vi "MotionProfile.vi"() -> ()   [LabVIEW 2016]
uses:
  <vilib>/Analysis/polynomials.llb/Polynomial Plot (Range).vi
  <vilib>/Analysis/polynomials.llb/nth Derivative of Polynomial (DBL).vi
  <vilib>/Analysis/NI_AALPro.lvlib
  <vilib>/addons/control/pid/NI_PID_pid.lvlib
panel:
  in  "Curve Constraints":cluster{"Orientiation Control":dbl, "Alpha":dbl}
  in  "Motion Constraints":T1={"Time Resolution (ms)"=10, "Max Acceleration"=40.0, "Cruising Velocity"=20.0}
  out "XY Graph 2":cluster{"X":dbl, "Y":dbl}[](graph)
  out "XY Graph":cluster{"X":dbl, "Y":dbl}[](graph)
  out "Corrected Motion Cluster":T2(array[cluster])
  in  "Velocity":dbl[](array[numeric])
  in  "Heading":dbl[](array[numeric])
  in  "X":dbl[](array[numeric])
  in  "Y":dbl[](array[numeric])
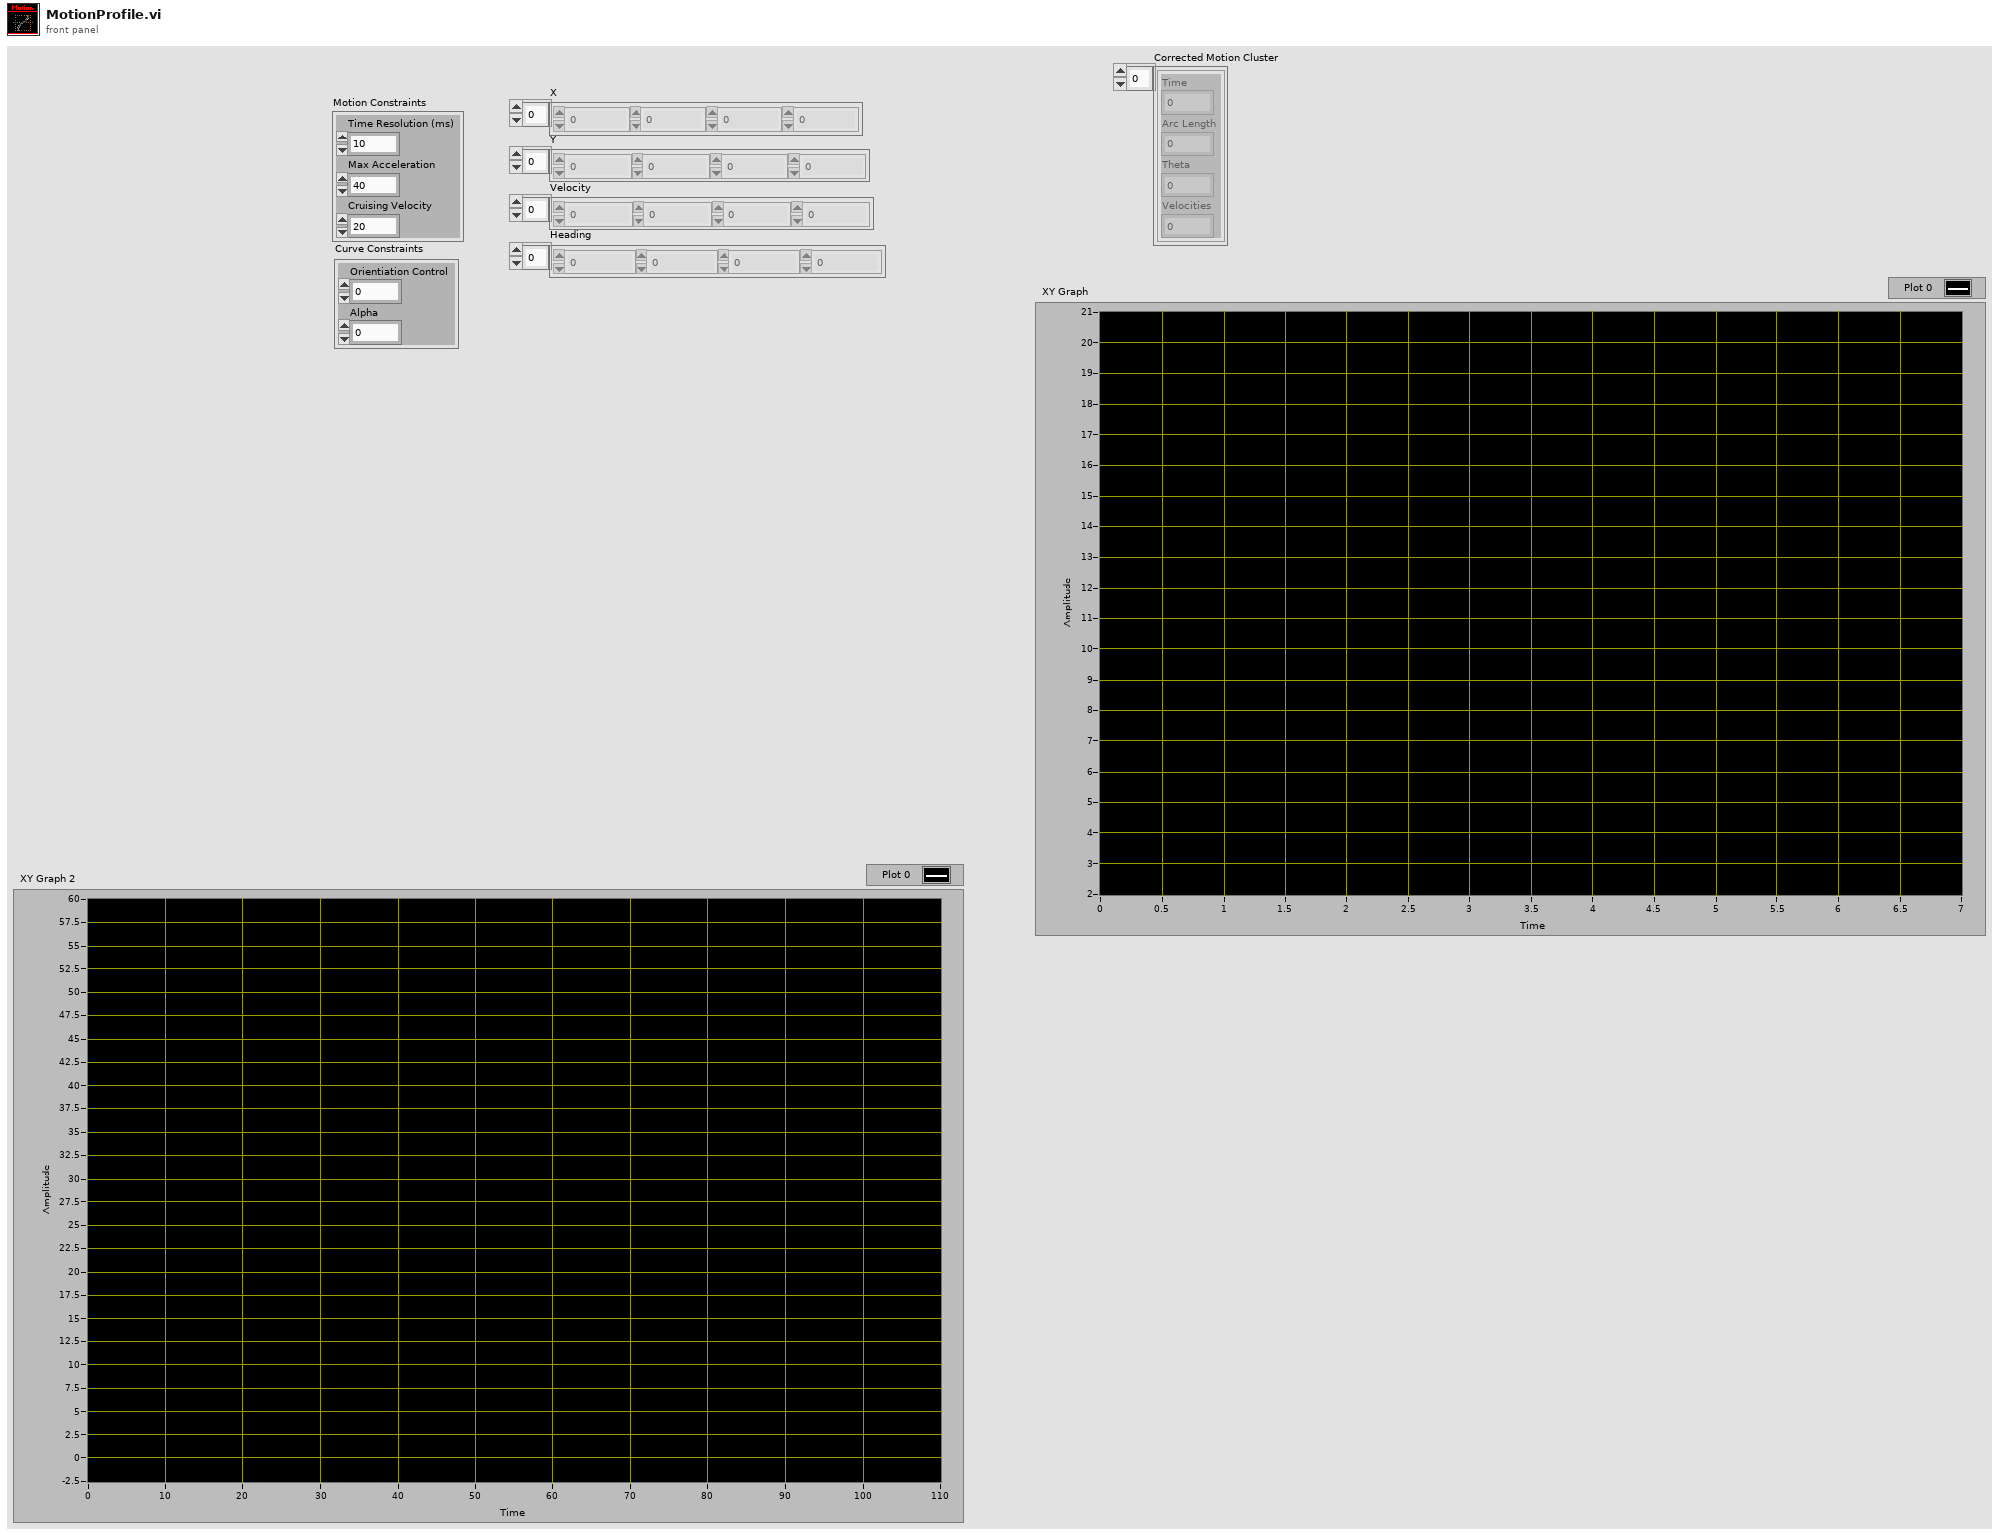
[diagram p1: front panel]
types:
  T1 = cluster{"Time Resolution (ms)":i32, "Max Acceleration":dbl, "Cruising Velocity":dbl}
  T2 = cluster{"Time":dbl, "Arc Length":dbl, "Theta":dbl, "Velocities":dbl}[]
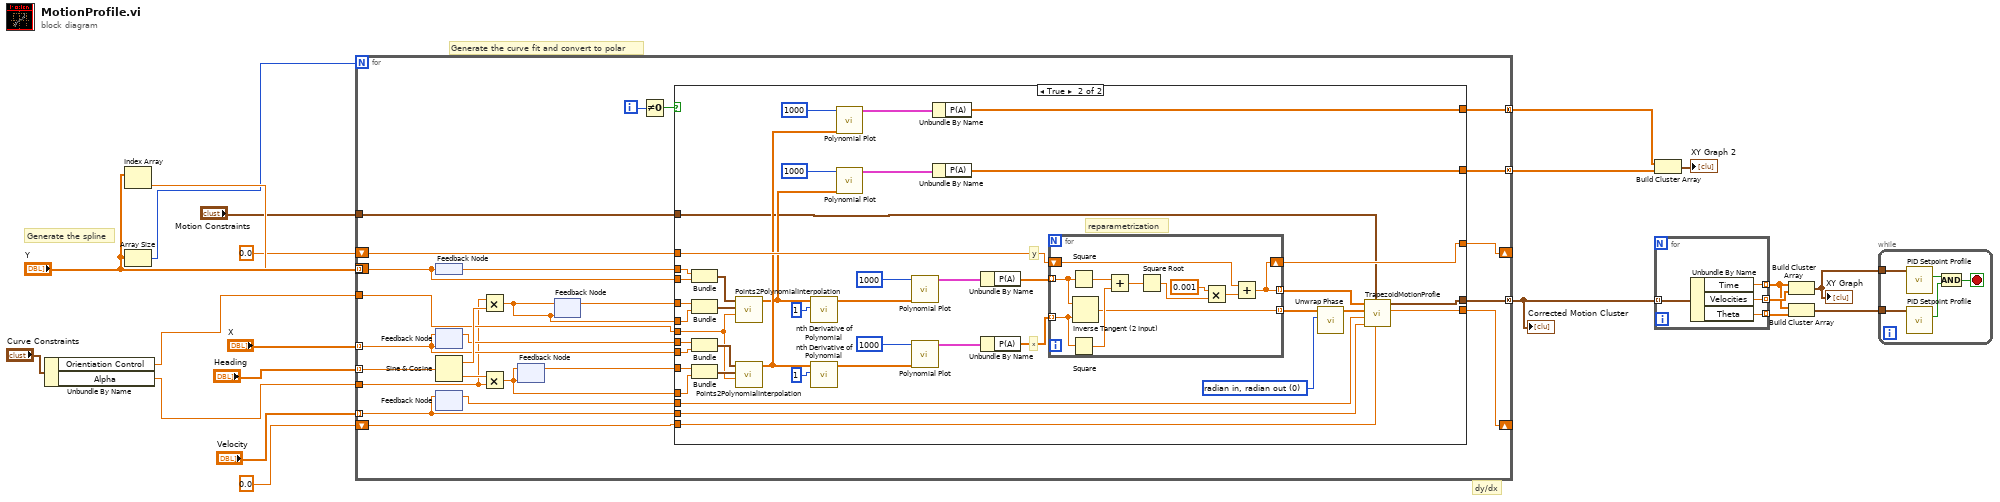
[diagram p0: block diagram]
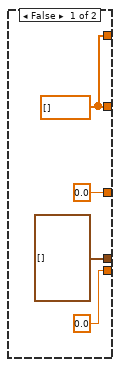
[diagram p2: hidden frame]
diagram:
  # "Generate the curve fit and convert to polar"
  # "dy/dx"
  # "Generate the spline"
  n1 = Unbundle By Name("Curve Constraints") -> ("Orientiation Control"=w2:dbl, "Alpha"=w1:dbl)
  n2 = Index Array(array="Y") -> (element=w17:dbl)  [unwired: 1 in]
  n3 = Array Size(array="Y") -> (size(s)=w16:i32)
  n4 = for {
    N: w16 -> [_]
    tunnel: "Y" -> [w38] mode=indexing
    tunnel: "Heading" -> [w46] mode=indexing
    tunnel: "X" -> [w34] mode=indexing
    tunnel: "Velocity" -> [w24] mode=indexing
    border: w17 -> [_]
    tunnel: w2 -> [w37]
    shift-right: [w33] -> _
    shift-left: 0.0 -> [w32]
    tunnel: [w30] -> w14 mode=concatenating
    shift-right: [w28] -> _
    shift-left: 0.0 ("Final Time") -> [w27]
    tunnel: [w26] -> w9 mode=concatenating
    tunnel: [w25] -> w10 mode=concatenating
    tunnel: w1 -> [w23]
    tunnel: "Motion Constraints" -> [w22]
    i -> [w29]
    n5 = feedback-in #1(w38) -> ()
    n6 = feedback #1() -> (w39:dbl)
    n7 = feedback #2(w34) -> (w40:dbl)
    n8 = feedback-in #2(w34) -> ()
    n9 = Sine & Cosine(0:w46) -> (1:w45:dbl, 2:w44:dbl)
    n10 = feedback #3() -> (w31:dbl)  [unwired: 1 in]
    n11 = feedback-in #3(w24) -> ()
    n12 = Multiply(x=w23, y=w45) -> (x*y=w36:dbl)
    n13 = Multiply(x=w44, y=w23) -> (x*y=w35:dbl)
    n14 = feedback #4(w35) -> (w42:dbl)
    n15 = feedback-in #4(w35) -> ()
    n16 = feedback #5(w36) -> (w41:dbl)
    n17 = feedback-in #5(w36) -> ()
    n18 = Not Equal To 0?(x=w29) -> (x != 0?=w43:bool)
    n19 = case shown="True" w43 {
      tunnel: w35 -> [_ w89]
      tunnel: w42 -> [_ w90]
      tunnel: w36 -> [_ w86]
      tunnel: w41 -> [_ w87]
      tunnel: w34 -> [_ w93]
      tunnel: w40 -> [_ w92]
      tunnel: w39 -> [_ w84]
      tunnel: w38 -> [_ w83]
      tunnel: w37 -> [_ w81]
      tunnel: [0.0 w72] -> w33
      tunnel: w32 -> [_ w71]
      tunnel: w24 -> [_ w66]
      tunnel: w31 -> [_ w65]
      tunnel: [T2 [] ("Corrected Motion Cluster") w64] -> w30
      tunnel: [0.0 ("Final Time") w63] -> w28
      tunnel: w27 -> [_ w62]
      tunnel: [w47 w52] -> w26
      tunnel: [w47 w54] -> w25
      tunnel: w22 -> [_ w51]
      frame False {
        w47 = dbl[] [] ("P(A)")
      }
      frame True {
        w70 = 0 items=["radian in, radian out", "radian in, degree out", "degree in, degree out", "degree in, radian out"] ("phase unit")
        # "reparametrization"
        # "x"
        # "y"
        n20 = Bundle("Numeric"=w84, "Numeric"=w83) -> (w82:cluster{"Numeric":dbl, "Numeric":dbl})  [unwired: 1 in]
        n21 = Bundle(w87, w86) -> (w85:cluster{dbl, dbl})  [unwired: 1 in]
        n22 = Bundle("Numeric"=w92, "Numeric"=w93) -> (w91:cluster{"Numeric":dbl, "Numeric":dbl})  [unwired: 1 in]
        n23 = Bundle(w90, w89) -> (w88:cluster{dbl, dbl})  [unwired: 1 in]
        n24 = call "Points2PolynomialInterpolation.vi"("Alpha Value"=w81, "Velocities"=w85, "Positions"=w82) -> ("Polynomial Coefficients (final = leading)"=w56:dbl[])  [unwired: 8 in]
        n25 = call "Points2PolynomialInterpolation.vi"("Alpha Value"=w81, "Velocities"=w88, "Positions"=w91) -> ("Polynomial Coefficients (final = leading)"=w57:dbl[])  [unwired: 8 in]
        n26 = call-poly <vilib>:"nth Derivative of Polynomial.vi"("order"=1, "P(x)"=w56) -> ("Nth Derivative of P(x)"=w76:dbl[])  [unwired: 8 in, 1 out]
        n27 = call-poly <vilib>:"nth Derivative of Polynomial.vi"("order"=1, "P(x)"=w57) -> ("Nth Derivative of P(x)"=w74:dbl[])  [unwired: 8 in, 1 out]
        n28 = call-poly <vilib>:"Polynomial Plot.vi"("P(x)"=w57, "samples"=1000) -> ("polynomial plot"=w53:cluster{"Ramp Pattern":dbl[], "P(A)":dbl[]})  [unwired: 8 in, 1 out]
        n29 = call-poly <vilib>:"Polynomial Plot.vi"("P(x)"=w56, "samples"=1000) -> ("polynomial plot"=w55:cluster{"Ramp Pattern":dbl[], "P(A)":dbl[]})  [unwired: 8 in, 1 out]
        n30 = call-poly <vilib>:"Polynomial Plot.vi"("P(x)"=w76, "samples"=1000) -> ("polynomial plot"=w77:cluster{"Ramp Pattern":dbl[], "P(A)":dbl[]})  [unwired: 8 in, 1 out]
        n31 = call-poly <vilib>:"Polynomial Plot.vi"("P(x)"=w74, "samples"=1000) -> ("polynomial plot"=w73:cluster{"Ramp Pattern":dbl[], "P(A)":dbl[]})  [unwired: 8 in, 1 out]
        n32 = Unbundle By Name(w53) -> ("P(A)"=w52:dbl[])
        n33 = Unbundle By Name(w55) -> ("P(A)"=w54:dbl[])
        n34 = Unbundle By Name(w77) -> ("P(A)"=w60:dbl[])
        n35 = Unbundle By Name(w73) -> ("P(A)"=w61:dbl[])
        n36 = for {
          shift-right: [w99] -> w72
          shift-left: w71 -> [w100]
          tunnel: [w99] -> w68 mode=indexing
          tunnel: [w98] -> w69 mode=indexing
          tunnel: w60 -> [w95] mode=indexing
          tunnel: w61 -> [w94] mode=indexing
          n37 = Square(x=w95) -> (x^2=w104:dbl)
          n38 = Square(x=w94) -> (x^2=w103:dbl)
          n39 = Inverse Tangent (2 Input)(1:w94, 2:w95) -> (0:w98:dbl)
          n40 = Add(x=w104, y=w103) -> (x+y=w102:dbl)
          n41 = Square Root(x=w102) -> (sqrt(x)=w101:dbl)
          n42 = Multiply(x=0.001, y=w101) -> (x*y=w97:dbl)
          n43 = Add(x=w100, y=w97) -> (x+y=w99:dbl)
        }
        n44 = call <vilib>:"Unwrap Phase.vi"("phase unit"=w70, "Phase"=w69) -> ("Unwrapped Phase"=w67:dbl[])  [unwired: 8 in, 1 out]
        n45 = call "TrapezoidMotionProfie.vi"("Start Time"=w62, "Constraints"=w51, "Final Velocity"=w66, "Initial Velocity"=w65, "Theta"=w67, "Arc Length"=w68) -> ("Final Time"=w63:dbl, "Motion Cluster"=w64:T2)  [unwired: 4 in]
      }
    }
  }
  "Corrected Motion Cluster" <- w14
  n46 = Build Cluster Array(w9, w10) -> (→"XY Graph 2":cluster{"p(x)":dbl, "p(x)":dbl}[])
  n47 = for {
    tunnel: w14 -> [w108] mode=indexing
    tunnel: [w107] -> w7 mode=indexing
    tunnel: [w106] -> w13 mode=indexing
    tunnel: [w105] -> w6 mode=indexing
    n48 = Unbundle By Name(w108) -> ("Time"=w107:dbl, "Velocities"=w106:dbl, "Theta"=w105:dbl)
  }
  n49 = Build Cluster Array(w7, w13) -> (w8:cluster{"Time":dbl, "Velocities":dbl}[])
  "XY Graph" <- w8
  n50 = Build Cluster Array(w7, w6) -> (w5:cluster{"Time":dbl, "Theta":dbl}[])
  n51 = while {
    tunnel: w8 -> [w113]
    tunnel: w5 -> [w112]
    stop <- w111 stop-if-true
    n52 = call <vilib>:"PID Setpoint Profile.vi"("setpoint profile"=w113) -> ("profile complete?"=w109:bool)  [unwired: 5 in, 3 out]
    n53 = call <vilib>:"PID Setpoint Profile.vi"("setpoint profile"=w112) -> ("profile complete?"=w110:bool)  [unwired: 5 in, 3 out]
    n54 = And(x=w109, y=w110) -> (x .and. y?=w111:bool)
  }
